vi "Pulse Stretch & Delay.vi"(1 "Delay (sec)":dbl, 2 "In":bool, 4 "Width (sec)":dbl=0.01) -> (5 "Out":bool)   [LabVIEW 2011]
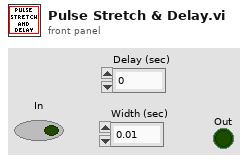
[diagram p1: front panel]
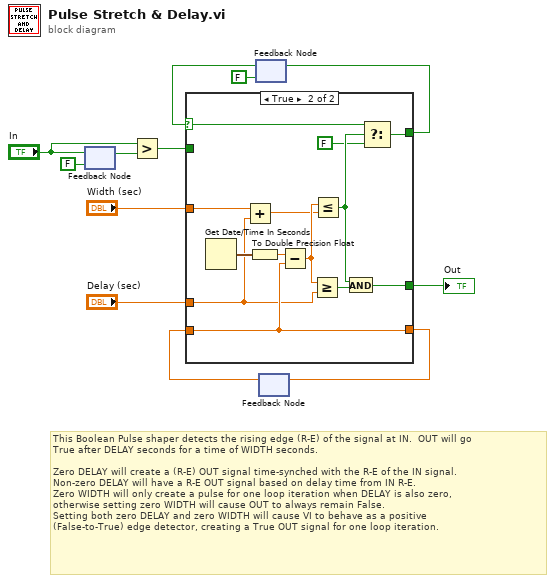
[diagram p0: block diagram]
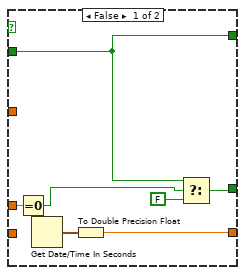
[diagram p2: hidden frame]
diagram:
  # "This Boolean Pulse shaper detects the rising edge (R-E) of the signal at IN.  OUT will go\nTrue after DELAY seconds for a time of WIDTH seconds. \n\nZero DELAY will create a (R-E) OUT signal time-synched with the R-E of the IN signal.\nNon-zero DELAY will have a R-E OUT signal based on delay time from IN R-E.\nZero WIDTH will only create a pulse for one loop iteration when DELAY is also zero,\notherwise setting zero WIDTH will cause OUT to always remain False.\nSetting both zero DELAY and zero WIDTH will cause VI to behave as a positive\n(False-to-True) edge detector, creating a True OUT signal for one loop iteration."
  n1 = feedback #1(FALSE ("input")) -> (w11:bool)
  n2 = feedback-in #1("In") -> ()
  n3 = Greater?(x="In", y=w11) -> (0:w2:bool)
  n4 = feedback #2(FALSE) -> (w6:bool)
  n5 = feedback #3() -> (w8:dbl)  [unwired: 1 in]
  n6 = case shown="True" w6 {
    selector: w6 -> [_ w23]
    tunnel: [w18 w27] -> w9
    tunnel: w8 -> [_ w27]
    tunnel: [w16 w31] -> w7
    tunnel: w2 -> [w16 _]
    tunnel: [w15 w28] -> w1
    tunnel: "Delay (sec)" -> [w17 w21]
    tunnel: "Width (sec)" -> [_ w20]
    frame False {
      n7 = Equal To 0?(x=w17) -> (x = 0?=w13:bool)
      n8 = Get Date/Time In Seconds() -> (seconds since 1Jan1904=w19:timestamp)
      n9 = To Double Precision Float(number=w19) -> (double precision float=w18:dbl)
      n10 = Select(t=w16, s=w13, f=FALSE) -> (s? t:f=w15:bool)
    }
    frame True {
      n11 = Get Date/Time In Seconds() -> (seconds since 1Jan1904=w32:timestamp)
      n12 = Add(x=w20, y=w21) -> (x+y=w25:dbl)
      n13 = To Double Precision Float(number=w32) -> (double precision float=w29:dbl)
      n14 = Subtract(x=w29, y=w27) -> (x-y=w26:dbl)
      n15 = Greater Or Equal?(x=w26, y=w21) -> (x >= y?=w30:bool)
      n16 = Less Or Equal?(x=w26, y=w25) -> (x <= y?=w24:bool)
      n17 = And(x=w24, y=w30) -> (x .and. y?=w28:bool)
      n18 = Select(t=w23, s=w24, f=FALSE) -> (s? t:f=w31:bool)
    }
  }
  "Out" <- w1
  n19 = feedback-in #2(w7) -> ()
  n20 = feedback-in #3(w9) -> ()
